vi "thcd_get_chan.vi"(6 "err_in":errorcluster, 7 "thcd_visa":refnum<visa-resource-name>, 9 "thcd_ch":T1=enum."1", 10 "thcd_b2r":u32, 11 "thcd_delay":u32=500) -> (0 "thcd_st":bool, 2 "thcd_res_str":string, 3 "thcd_res":T2, 4 "err_out":errorcluster, 5 "thcd_visa":refnum<visa-resource-name>)   [LabVIEW 2020]
uses:
  mks946_controls/ctrl_chn_thcd.ctl
panel:
  out "mks946_resp":string
  out "mks946_val":dbl
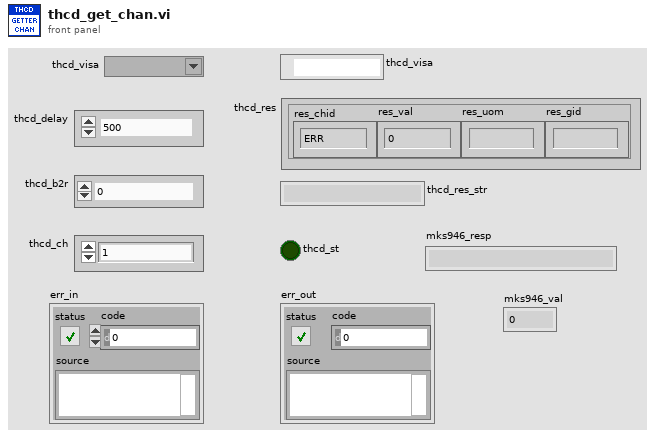
[diagram p1: front panel]
types:
  T1 = typedef "ctrl_chn_thcd.ctl" = enum8{"ERR", "1", "2", "3", "4"}
  T2 = cluster{"res_chid":T1, "res_val":dbl, "res_uom":string, "res_gid":string}
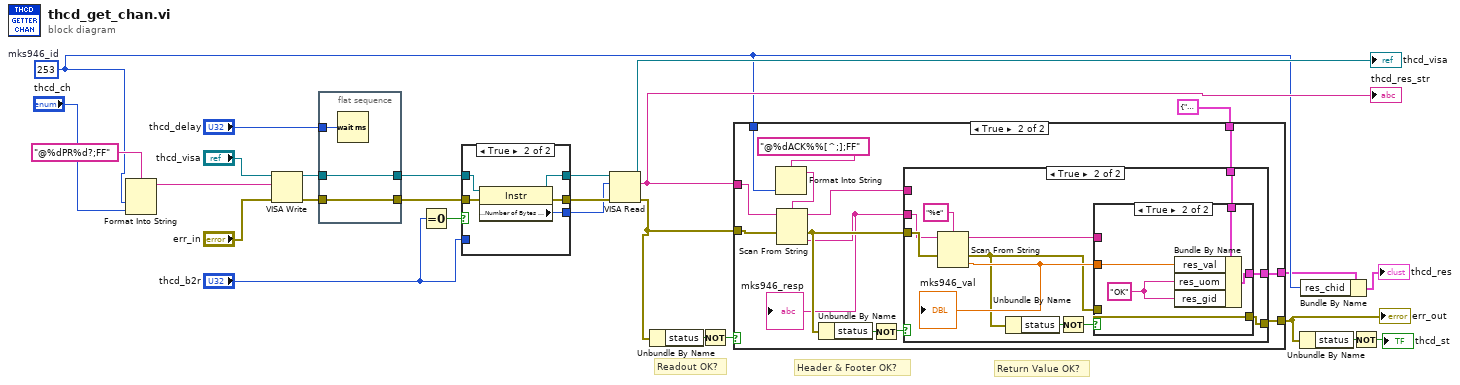
[diagram p0: block diagram]
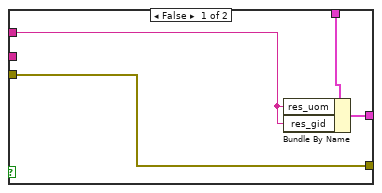
[diagram p4: hidden frame]
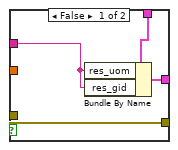
[diagram p5: hidden frame]
diagram:
  w3 = 253  # mks946_id
  # "Return Value OK?"
  # "Header & Footer OK?"
  # "Readout OK?"
  n1 = Format Into String(format string="@%dPR%d?;FF", w3, "thcd_ch") -> (resulting string=w22:string)  [unwired: 2 in, 1 out]
  n2 = VISA Write(VISA resource name="thcd_visa", write buffer=w22, error in (no error)="err_in") -> (VISA resource name out=w26:refnum<visa-resource-name>, error out=w27:errorcluster)  [unwired: 1 out]
  n3 = flat-sequence {
    tunnel: w27 -> [w29]
    tunnel: [w29] -> w16
    tunnel: w26 -> [w28]
    tunnel: [w28] -> w17
    tunnel: "thcd_delay" -> [w30]
    frame #0 {
      n4 = Wait (ms)(milliseconds to wait=w30) -> ()  [unwired: 1 out]
    }
  }
  n5 = Equal To 0?(x="thcd_b2r") -> (x = 0?=w18:bool)
  n6 = case shown="True" w18 {
    tunnel: [w32 w38] -> w15
    tunnel: [w31 w37] -> w14
    tunnel: [w33 w36] -> w13
    tunnel: "thcd_b2r" -> [w33 _]
    tunnel: w17 -> [w32 w35]
    tunnel: w16 -> [w31 w34]
    frame False {
    }
    frame True {
      n7 = property class="Instr"(reference=w35, error in=w34) -> (reference out=w38:refnum<visa-resource-name>, error out=w37:errorcluster, "Serial Settings:Number of Bytes at Serial Port"=w36:u32)
    }
  }
  n8 = VISA Read(VISA resource name=w15, byte count=w13, error in (no error)=w14) -> (VISA resource name out=→"thcd_visa":refnum<visa-resource-name>, read buffer=w8:string, error out=w7:errorcluster)  [unwired: 1 out]
  "thcd_res_str" <- w8
  n9 = Unbundle By Name(w7) -> ("status"=w19:bool)
  n10 = Not(x=w19) -> (.not. x?=w9:bool)
  n11 = case shown="True" w9 {
    tunnel: [w39 w42] -> w4
    tunnel: T2 {"res_chid"=enum."ERR", "res_val"=0.0, "res_uom"="", "res_gid"=""} ("thcd_res 2") -> [w40 w44]
    tunnel: [w40 w43] -> w2
    tunnel: w8 -> [_ w53]
    tunnel: w7 -> [w39 w52]
    tunnel: w3 -> [_ w51]
    frame False {
    }
    frame True {
      n12 = Format Into String(format string="@%dACK%%[^;];FF", w51) -> (resulting string=w50:string)  [unwired: 2 in, 1 out]
      n13 = Scan From String(format string=w50, input string=w53, error in=w52) -> (remaining string=w41:string, error out=w46:errorcluster, output 1=w45:string)  [unwired: 2 in, 1 out]
      "mks946_resp" <- w45
      n14 = Unbundle By Name(w46) -> ("status"=w48:bool)
      n15 = Not(x=w48) -> (.not. x?=w47:bool)
      n16 = case shown="True" w47 {
        tunnel: w46 -> [w57 w67]
        tunnel: w45 -> [_ w66]
        tunnel: w44 -> [w55 w64]
        tunnel: [w56 w62] -> w43
        tunnel: [w57 w59] -> w42
        tunnel: w41 -> [w54 _]
        frame False {
          n17 = Bundle By Name(cluster=w55, "res_uom"=w54, "res_gid"=w54) -> (w56:T2)
        }
        frame True {
          n18 = Scan From String(format string="%e", input string=w66, error in=w67) -> (remaining string=w58:string, error out=w60:errorcluster, output 1=w63:dbl)  [unwired: 2 in, 1 out]
          "mks946_val" <- w63
          n19 = Unbundle By Name(w60) -> ("status"=w65:bool)
          n20 = Not(x=w65) -> (.not. x?=w61:bool)
          n21 = case shown="True" w61 {
            tunnel: w64 -> [w70 w77]
            tunnel: w63 -> [_ w76]
            tunnel: [w71 w74] -> w62
            tunnel: w60 -> [w72 w73]
            tunnel: [w72 w73] -> w59
            tunnel: w58 -> [w69 _]
            frame False {
              n22 = Bundle By Name(cluster=w70, "res_uom"=w69, "res_gid"=w69) -> (w71:T2)
            }
            frame True {
              w75 = "OK"
              n23 = Bundle By Name(cluster=w77, "res_val"=w76, "res_uom"=w75, "res_gid"=w75) -> (w74:T2)
            }
          }
        }
      }
    }
  }
  "err_out" <- w4
  n24 = Unbundle By Name(w4) -> ("status"=w6:bool)
  n25 = Bundle By Name(cluster=w2, "res_chid"=w3) -> (→"thcd_res":T2)
  n26 = Not(x=w6) -> (.not. x?=→"thcd_st":bool)
